vi "DSF.Engine.Transceiver Thread.Transfer Group.Build.vi"(8 "error in (no error)":errorcluster, 10 "Transfer Group in":refnum<class "DSF.Engine.Transfer Group.lvclass">, 11 "Transceiver Thread in":refnum<class "DSF.Engine.Transceiver Thread.lvclass">) -> (0 "error out":errorcluster, 2 "Transfer Group out":refnum<class "DSF.Engine.Transfer Group.lvclass">, 3 "Transceiver Thread out":refnum<class "DSF.Engine.Transceiver Thread.lvclass">)   [LabVIEW 2017, in "DSF.Engine.lvlib" / "DSF.Engine.Transceiver Thread.lvclass"]
uses:
  DSF.Engine.Transceiver Thread.lvclass
  Transfer/DSF.Engine.Transfer Group.lvclass
  Transfer/DSF.Engine.Transfer Group.lvclass/DSF.Engine.Transfer Group.ctl
  Transfer/DSF.Engine.Transfer.lvclass/DSF.Engine.Transfer.ctl
  DSF.Engine.Transceiver Thread.lvclass/DSF.Engine.Transceiver Thread.ctl
  Pointer/DSF.Engine.Pointer.DBL.lvclass/DSF.Engine.Pointer.DBL.ctl
  Buffer/DSF.Engine.Memory.Buffer.Insert Channels.Preserve Value.vi
  Transfer/DSF.Engine.Transfer.Get String Buffer.vi
  Transfer/DSF.Engine.Transfer.Get Intermediate Buffer.vi
  DSF.Engine.Transceiver Thread.Set Channels Buffer.vi
  DSF.Engine.Transceiver Thread.Get Channels Buffer.vi
  Transfer/DSF.Engine.Transfer.Get Channel Blocks.vi
  Pointer/DSF.Engine.Pointer.DBL.Read.vi
  Pointer/DSF.Engine.Pointer.DBL.Get Channel Count.vi
  Pointer/DSF.Engine.Pointer.DBL.lvclass
  C:/Git/DSF/DSF Core/Built/PharLap x86/Dependencies/c/Memory Manager.lvlibp/1abvi3w/vi.lib/National Instruments/Memory Manager/Classes/Pointer/Memory.Pointer.lvclass
  Buffer/DSF.Engine.Memory.Buffer.Write.vi
  Buffer/DSF.Engine.Memory.Buffer.Write.1D.U64.vi
  Buffer/DSF.Engine.Memory.Buffer.Write.1D.U32.vi
  Buffer/DSF.Engine.Memory.Buffer.Write.1D.U16.vi
  Buffer/DSF.Engine.Memory.Buffer.Write.1D.U8.vi
  Buffer/DSF.Engine.Memory.Buffer.Write.1D.I64.vi
  Buffer/DSF.Engine.Memory.Buffer.Write.1D.I32.vi
  Buffer/DSF.Engine.Memory.Buffer.Write.1D.I16.vi
  Buffer/DSF.Engine.Memory.Buffer.Write.1D.I8.vi
  Buffer/DSF.Engine.Memory.Buffer.Write.1D.DBL.vi
  Buffer/DSF.Engine.Memory.Buffer.Write.1D.SGL.vi
  Buffer/DSF.Engine.Memory.Buffer.Write.1D.Bool.vi
  Built/Core/Memory Manager.lvlibp/1abvi3w/vi.lib/National Instruments/Memory Manager/Classes/Pointer/Memory.Pointer.Read.vi
  Built/Core/Memory Manager.lvlibp/1abvi3w/vi.lib/National Instruments/Memory Manager/Classes/Pointer/Memory.Pointer.Read.1D.DBL.vi
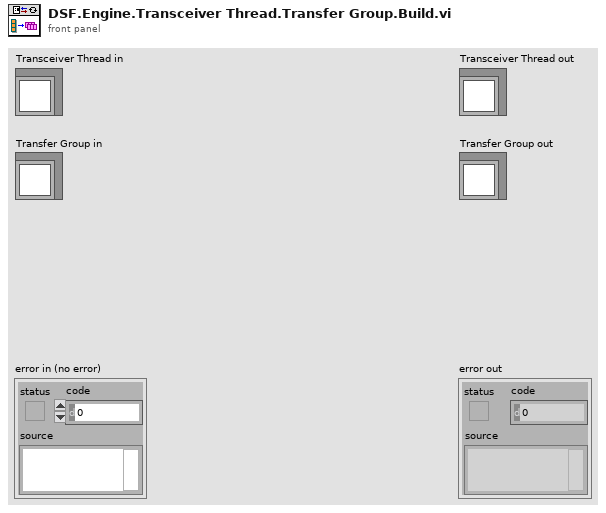
[diagram p1: front panel]
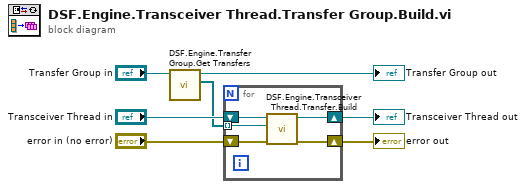
[diagram p0: block diagram]
diagram:
  n1 = call "DSF.Engine.Transfer Group.Get Transfers.vi"("Transfer Group in"="Transfer Group in") -> ("Transfers"=w5:refnum<class "DSF.Engine.Transfer.lvclass">[], "Transfer Group out"=→"Transfer Group out":refnum<class "DSF.Engine.Transfer Group.lvclass">)  [unwired: 9 in]
  n2 = for {
    tunnel: w5 -> [w8] mode=indexing
    shift-right: [w9] -> w4
    shift-left: "Transceiver Thread in" -> [w10]
    shift-right: [w11] -> w3
    shift-left: "error in (no error)" -> [w12]
    n3 = call "DSF.Engine.Transceiver Thread.Transfer.Build.vi"("error in (no error)"=w12, "Transfer"=w8, "Transceiver Thread in"=w10) -> ("error out"=w11:errorcluster, "Transceiver Thread out"=w9:refnum<class "DSF.Engine.Transceiver Thread.lvclass">)  [unwired: 7 in]
  }
  "error out" <- w3
  "Transceiver Thread out" <- w4
